vi "gmailALT.vi"(0 "Para: (nome)":string, 1 "Para: (endereço)":string, 2 "De: (nome)":string, 3 "Assunto":string="ALARME", 4 "Senha da Conta - GMAIL":string, 5 "Mensagem":string, 6 "Conta Criada no GMAIL":string, 7 "Anexar Arquivo (caminho)":path, 8 "De: (endereço)":string) -> ()   [LabVIEW 2018]
panel:
  out "error out":errorcluster
  in  "Cópia para":string
  in  "Port":i32=587
  in  "Enable SSL":bool=TRUE
  in  "Endereço SMTP - Gmail":string="smtp.gmail.com"
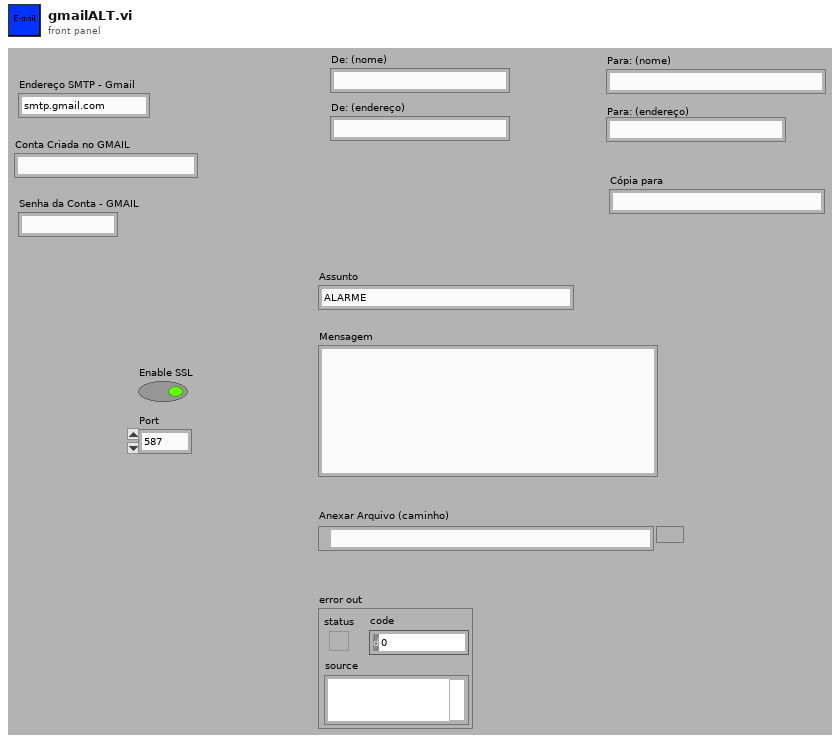
[diagram p1: front panel]
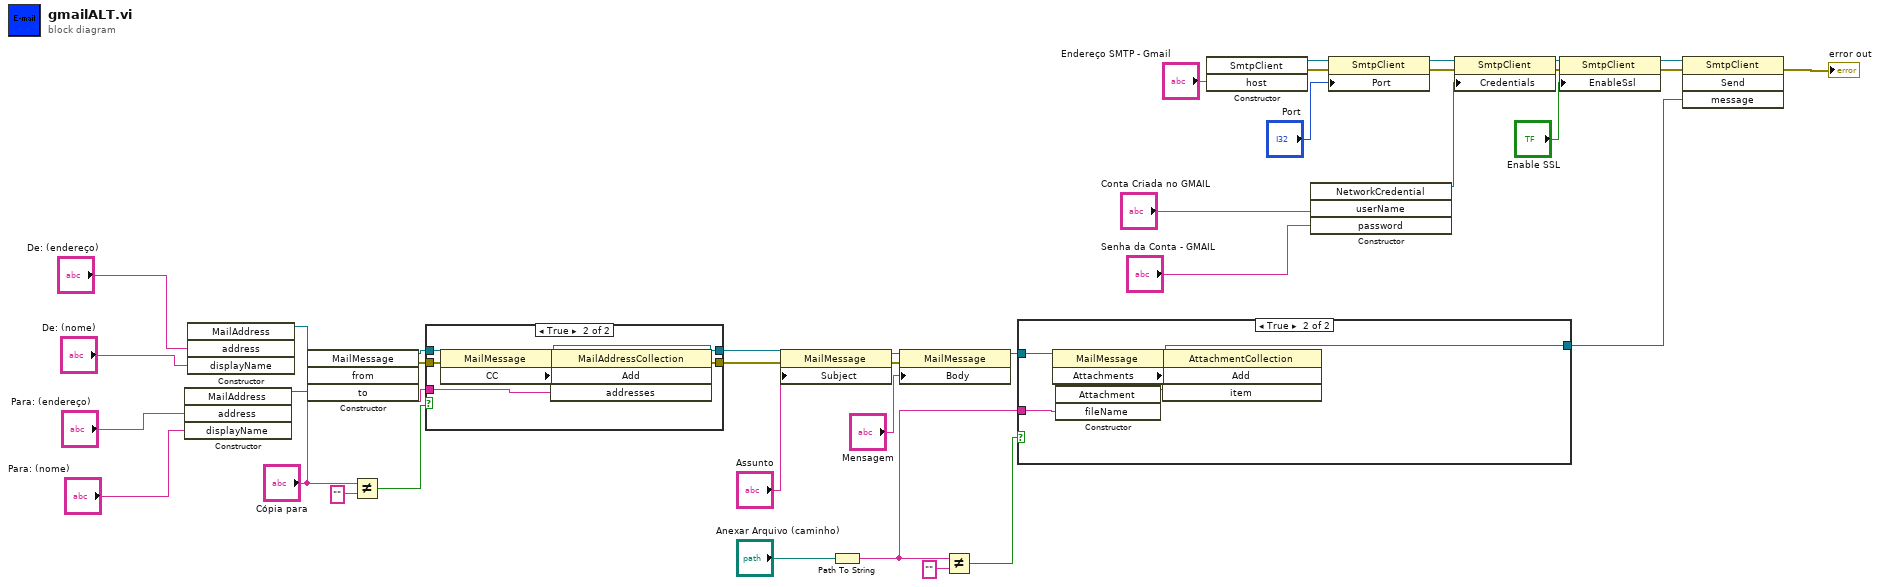
[diagram p0: block diagram]
diagram:
  n1 = constructor class="MailAddress"("address"="Para: (endereço)", "displayName"="Para: (nome)") -> (reference out=w38:refnum<k24>)  [unwired: 3 in, 4 out]
  n2 = constructor class="MailAddress"("address"="De: (endereço)", "displayName"="De: (nome)") -> (reference out=w37:refnum<k24>)  [unwired: 3 in, 4 out]
  n3 = constructor class="MailMessage"("from"=w37, "to"=w38) -> (reference out=w5:refnum<k24>, error out=w4:errorcluster)  [unwired: 3 in, 3 out]
  n4 = Not Equal?(x="Cópia para", y="") -> (x != y?=w7:bool)
  n5 = case shown="True" w7 {
    tunnel: "Cópia para" -> [_ w45]
    tunnel: w5 -> [w40 w44]
    tunnel: w4 -> [w39 w43]
    tunnel: [w40 w42] -> w3
    tunnel: [w39 w41] -> w2
    frame False {
    }
    frame True {
      n6 = property class="MailMessage"(reference=w44, error in=w43) -> (reference out=w42:refnum<k24>, error out=w47:errorcluster, "CC"=w46:refnum<k24>)
      n7 = invoke class="MailAddressCollection" method="Add"(reference=w46, error in=w47, "addresses"=w45) -> (error out=w41:errorcluster)  [unwired: 1 in, 3 out]
    }
  }
  n8 = property class="MailMessage"(reference=w3, error in=w2, "Subject"="Assunto") -> (reference out=w28:refnum<k24>, error out=w36:errorcluster)
  n9 = Path To String(path="Anexar Arquivo (caminho)") -> (string=w9:string)
  n10 = property class="MailMessage"(reference=w28, error in=w36, "Body"="Mensagem") -> (reference out=w14:refnum<k24>)  [unwired: 1 out]
  n11 = Not Equal?(x=w9, y="") -> (x != y?=w10:bool)
  n12 = case shown="True" w10 {
    tunnel: w14 -> [w48 w51]
    tunnel: [w48 w50] -> w13
    tunnel: w9 -> [_ w49]
    frame False {
    }
    frame True {
      n13 = property class="MailMessage"(reference=w51) -> (reference out=w50:refnum<k24>, error out=w54:errorcluster, "Attachments"=w52:refnum<k24>)  [unwired: 1 in]
      n14 = constructor class="Attachment"("fileName"=w49) -> (reference out=w53:refnum<k24>)  [unwired: 3 in, 3 out]
      n15 = invoke class="AttachmentCollection" method="Add"(reference=w52, error in=w54, "item"=w53) -> ()  [unwired: 1 in, 4 out]
    }
  }
  n16 = constructor class="SmtpClient"("host"="Endereço SMTP - Gmail") -> (reference out=w22:refnum<k24>, error out=w18:errorcluster)  [unwired: 3 in, 2 out]
  n17 = constructor class="NetworkCredential"("userName"="Conta Criada no GMAIL", "password"="Senha da Conta - GMAIL") -> (reference out=w23:refnum<k24>)  [unwired: 3 in, 4 out]
  n18 = property class="SmtpClient"(reference=w22, error in=w18, "Port"="Port") -> (reference out=w21:refnum<k24>, error out=w17:errorcluster)
  n19 = property class="SmtpClient"(reference=w21, error in=w17, "Credentials"=w23) -> (reference out=w20:refnum<k24>, error out=w16:errorcluster)
  n20 = property class="SmtpClient"(reference=w20, error in=w16, "EnableSsl"="Enable SSL") -> (reference out=w19:refnum<k24>, error out=w15:errorcluster)
  n21 = invoke class="SmtpClient" method="Send"(reference=w19, error in=w15, "message"=w13) -> (error out=→"error out":errorcluster)  [unwired: 1 in, 3 out]
